vi "Get_System_Error.vi"(8 "error in (no error)":errorcluster, 11 ".NET Reference in":refnum<k24>) -> (0 "error out":errorcluster, 2 "error":string, 3 "Reference out":refnum<k24>)   [LabVIEW 2017]
uses:
  D:/test/FULLband-sts/Fullband_Sample/DLL/InstrumentDLL.dll
  DLL/InstrumentDLL.dll
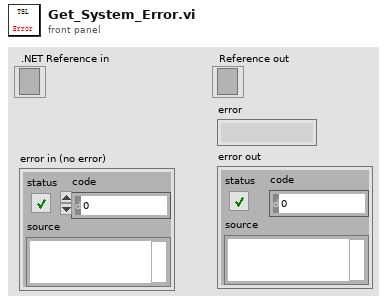
[diagram p1: front panel]
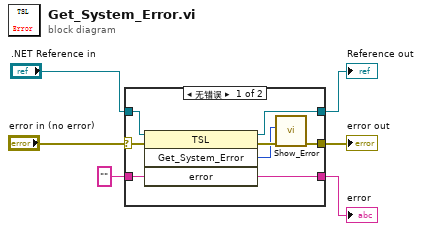
[diagram p0: block diagram]
diagram:
  n1 = case shown="无错误" "error in (no error)" {
    selector: "error in (no error)" -> [w7 w15]
    tunnel: [w14 w17] -> w2
    tunnel: ".NET Reference in" -> [w13 w16]
    tunnel: [w12 w16] -> w5
    tunnel: "" ("error") -> [w11 w17]
    tunnel: [w8 w15] -> w3
    frame No Error {
      n2 = invoke on="调用节点" class="TSL" method="Get_System_Error"(reference=w13, error in=w7, "error"=w11) -> (reference out=w12:refnum<k24>, error out=w10:errorcluster, "Get_System_Error"=w9:i32, "error"=w14:string)  [unwired: 1 in]
      n3 = call "Show_Error.vi"("error in (no error)"=w10, "Error"=w9) -> ("error out"=w8:errorcluster)  [unwired: 9 in]
    }
    frame Error {
    }
  }
  "error" <- w2
  "Reference out" <- w5
  "error out" <- w3
